vi "Fetch - NF.vi"(8 "error in":errorcluster, 11 "Refnum in":refnum<k21>) -> (0 "error out":errorcluster, 1 "Analyzer Noise Figure (dB)":dbl[][](array[numeric]), 2 "DUT Noise Figure (dB)":dbl[][](array[numeric]), 3 "Refnum out":refnum<k21>, 5 "Results":T1(array[cluster]))   [LabVIEW 2023]
uses:
  <vilib>/RFmx/SpecAn/mx/RFmxSpecAn.llb/RFmxSpecAn NF Fetch Y-Factors.vi
  <vilib>/RFmx/SpecAn/mx/RFmxSpecAn.llb/RFmxSpecAn NF Fetch Y-Factor Powers.vi
  <vilib>/RFmx/SpecAn/mx/RFmxSpecAn.llb/RFmxSpecAn NF Fetch Analyzer Noise Figure.vi
  <vilib>/RFmx/SpecAn/mx/RFmxSpecAn.llb/RFmxSpecAn NF Fetch DUT Noise Figure and Gain.vi
  <resource>/objmgr/RFmxSpecAn.rc
panel:
  out "Analyzer NF":T2
  out "DUT NF":T3
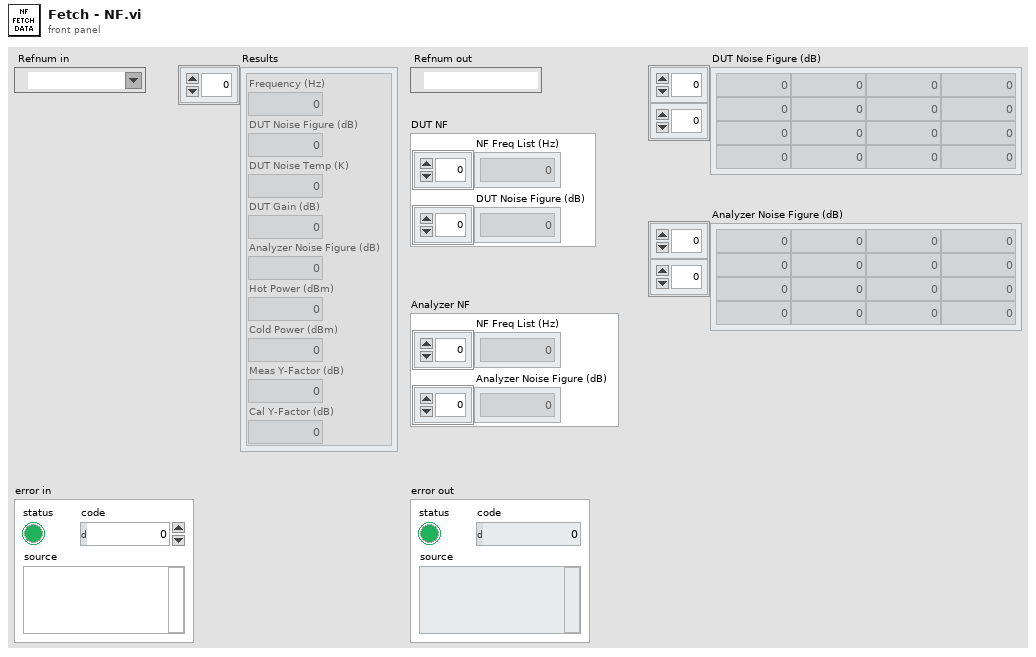
[diagram p1: front panel]
types:
  T1 = cluster{"Frequency (Hz)":dbl, "DUT Noise Figure (dB)":dbl, "DUT Noise Temp (K)":dbl, "DUT Gain (dB)":dbl, "Analyzer Noise Figure (dB)":dbl, "Hot Power (dBm)":dbl, "Cold Power (dBm)":dbl, "Meas Y-Factor (dB)":dbl, "Cal Y-Factor (dB)":dbl}[]
  T2 = cluster{"NF Freq List (Hz)":dbl[], "Analyzer Noise Figure (dB)":dbl[]}
  T3 = cluster{"NF Freq List (Hz)":dbl[], "DUT Noise Figure (dB)":dbl[]}
  T4 = cluster{"Frequency (Hz)":dbl, "DUT Noise Figure (dB)":dbl, "DUT Noise Temp (K)":dbl, "DUT Gain (dB)":dbl, "Analyzer Noise Figure (dB)":dbl, "Hot Power (dBm)":dbl, "Cold Power (dBm)":dbl, "Meas Y-Factor (dB)":dbl, "Cal Y-Factor (dB)":dbl}
  T5 = cluster{dbl[], "Analyzer Noise Figure (dB)":dbl[]}
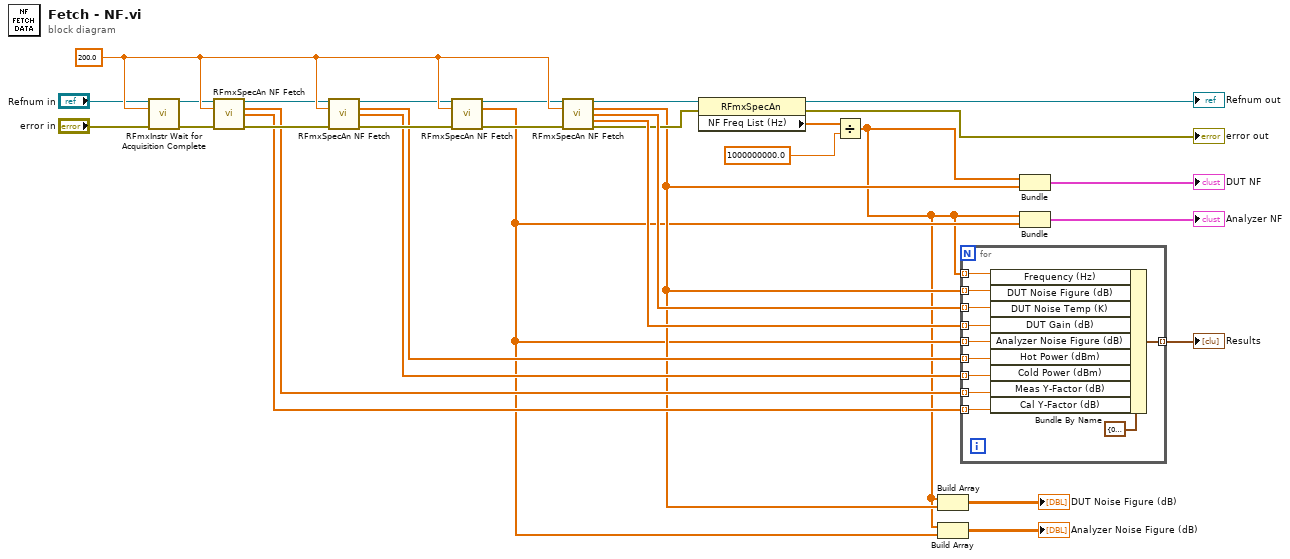
[diagram p0: block diagram]
diagram:
  w31 = 200.0 ("Timeout (s)")
  n1 = call <vilib>:"RFmxInstr Wait for Acquisition Complete.vi"("Instrument Handle In"="Refnum in", "Timeout (s)"=w31, "error in (no error)"="error in") -> ("Instrument Handle Out"=w29:refnum<k21>, "error out"=w30:errorcluster)  [unwired: 11 in]
  n2 = call-poly <vilib>:"RFmxSpecAn NF Fetch.vi"("Instrument Handle In"=w29, "Timeout (s)"=w31, "error in (no error)"=w30) -> ("Instrument Handle Out"=w23:refnum<k21>, "Measurement Y-Factor (dB)"=w20:dbl[], "Calibration Y-Factor (dB)"=w21:dbl[], "error out"=w24:errorcluster)  [unwired: 9 in]
  n3 = call-poly <vilib>:"RFmxSpecAn NF Fetch.vi"("Instrument Handle In"=w23, "Timeout (s)"=w31, "error in (no error)"=w24) -> ("Instrument Handle Out"=w25:refnum<k21>, "Hot Power (dBm)"=w19:dbl[], "Cold Power (dBm)"=w18:dbl[], "error out"=w26:errorcluster)  [unwired: 9 in]
  n4 = call-poly <vilib>:"RFmxSpecAn NF Fetch.vi"("Instrument Handle In"=w25, "Timeout (s)"=w31, "error in (no error)"=w26) -> ("Instrument Handle Out"=w27:refnum<k21>, "Analyzer Noise Figure (dB)"=w3:dbl[], "error out"=w28:errorcluster)  [unwired: 10 in]
  n5 = call-poly <vilib>:"RFmxSpecAn NF Fetch.vi"("Instrument Handle In"=w27, "Timeout (s)"=w31, "error in (no error)"=w28) -> ("Instrument Handle Out"=w14:refnum<k21>, "DUT Noise Figure (dB)"=w6:dbl[], "DUT Noise Temperature (K)"=w16:dbl[], "DUT Gain (dB)"=w17:dbl[], "error out"=w15:errorcluster)  [unwired: 8 in]
  n6 = property class="RFmxSpecAn"(reference=w14, error in=w15) -> (reference out=→"Refnum out":refnum<k21>, error out=→"error out":errorcluster, "NF Freq List (Hz)"=w4:dbl[])
  n7 = Divide(x=w4, y=1000000000.0 ("Timeout (s)")) -> (x/y=w2:dbl[])
  n8 = Build Array(w2, w6) -> (→"DUT Noise Figure (dB)":dbl[][])
  n9 = Build Array(w2, w3) -> (→"Analyzer Noise Figure (dB)":dbl[][])
  n10 = for {
    tunnel: w6 -> [w42] mode=indexing
    tunnel: w16 -> [w41] mode=indexing
    tunnel: w17 -> [w40] mode=indexing
    tunnel: w3 -> [w39] mode=indexing
    tunnel: w19 -> [w38] mode=indexing
    tunnel: w18 -> [w37] mode=indexing
    tunnel: w20 -> [w36] mode=indexing
    tunnel: w21 -> [w35] mode=indexing
    tunnel: [w34] -> w8 mode=indexing
    tunnel: w2 -> [w33] mode=indexing
    n11 = Bundle By Name(cluster=T4 {"Frequency (Hz)"=0.0, "DUT Noise Figure (dB)"=0.0, "DUT Noise Temp (K)"=0.0, "DUT Gain (dB)"=0.0, "Analyzer Noise Figure (dB)"=0.0, "Hot Power (dBm)"=0.0, "Cold Power (dBm)"=0.0, "Meas Y-Factor (dB)"=0.0, "Cal Y-Factor (dB)"=0.0} ("Common Results"), "Frequency (Hz)"=w33, "DUT Noise Figure (dB)"=w42, "DUT Noise Temp (K)"=w41, "DUT Gain (dB)"=w40, "Analyzer Noise Figure (dB)"=w39, "Hot Power (dBm)"=w38, "Cold Power (dBm)"=w37, "Meas Y-Factor (dB)"=w36, "Cal Y-Factor (dB)"=w35) -> (w34:T4)
  }
  "Results" <- w8
  n12 = Bundle(w2, "DUT Noise Figure (dB)"=w6) -> (→"DUT NF":cluster{dbl[], "DUT Noise Figure (dB)":dbl[]})  [unwired: 1 in]
  n13 = Bundle(w2, "Analyzer Noise Figure (dB)"=w3) -> (→"Analyzer NF":T5)  [unwired: 1 in]
